vi "mongo_cursor_bson.vi"(11 "cursor ptr":u32) -> (3 "bson ptr":u32)   [LabVIEW 2013]
uses:
  mongo-c-driver/libmongoc.so
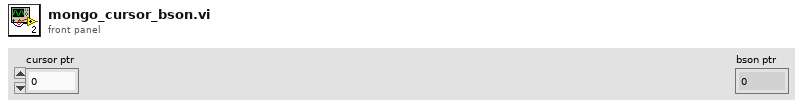
[diagram p1: front panel]
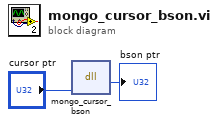
[diagram p0: block diagram]
diagram:
  n1 = dll-call lib="home/scot/dev/git/mongo-c-driver/libmongoc.so" fn="mongo_cursor_bson"("cursor ptr"="cursor ptr") -> ("bson ptr"=→"bson ptr":u32)  [unwired: 4 in, 2 out]
